vi "Routine.vi"(11 "Base Queue in":refnum<class "Base Queue.lvclass">) -> (3 "Base Queue out":refnum<class "Base Queue.lvclass">)   [LabVIEW 2021, in "jettl.lvlib" / "Base Queue.lvlib" / "Base Queue.lvclass"]
uses:
  Base Queue.lvclass
  Base Queue.lvclass/Base Queue.ctl
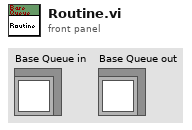
[diagram p1: front panel]
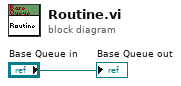
[diagram p0: block diagram]
diagram:
  "Base Queue out" <- "Base Queue in"
